vi "CompileCorrInfoNetDut.vi"(7 "Frame Direction":T1, 8 "error in (no error)":errorcluster, 10 "Frame Direction Prop":string, 11 "Device Item Ref in":T5 format="%.0x") -> (0 "error out":errorcluster, 2 "Corruption Info Network_DUT":T2 {"Frame Infos Array"."CRC Index" min=-7 max=7; "Frame Infos Array"."DLC Length  Corruption Index" min=-8 max=8}, 3 "Device Item Ref out":T5 format="%.0x")   [LabVIEW 2018, in "CAN Gateway System Explorer.lvlib"]
uses:
  CAN Gateway System Explorer.lvlib
  <vilib>/NI Veristand/Custom Device API/Custom Device Item Ref.ctl
  Shared/CTLs/Corruption Info.ctl
  Shared/CTLs/Frame.ctl
  Shared/CTLs/Signal_Data_Trigger.ctl
  Types/FrameDirection.ctl
  Types/FramesCluster.ctl
  <vilib>/NI Veristand/Custom Device API/Get Item Property (Variant).vi
  Shared/Constants.vi
  <vilib>/NI Veristand/Custom Device API/Get Item Property (String).vi
  <vilib>/NI Veristand/Custom Device API/Custom Device API.lvlib
  Shared/CAN Gateway Shared.lvlib
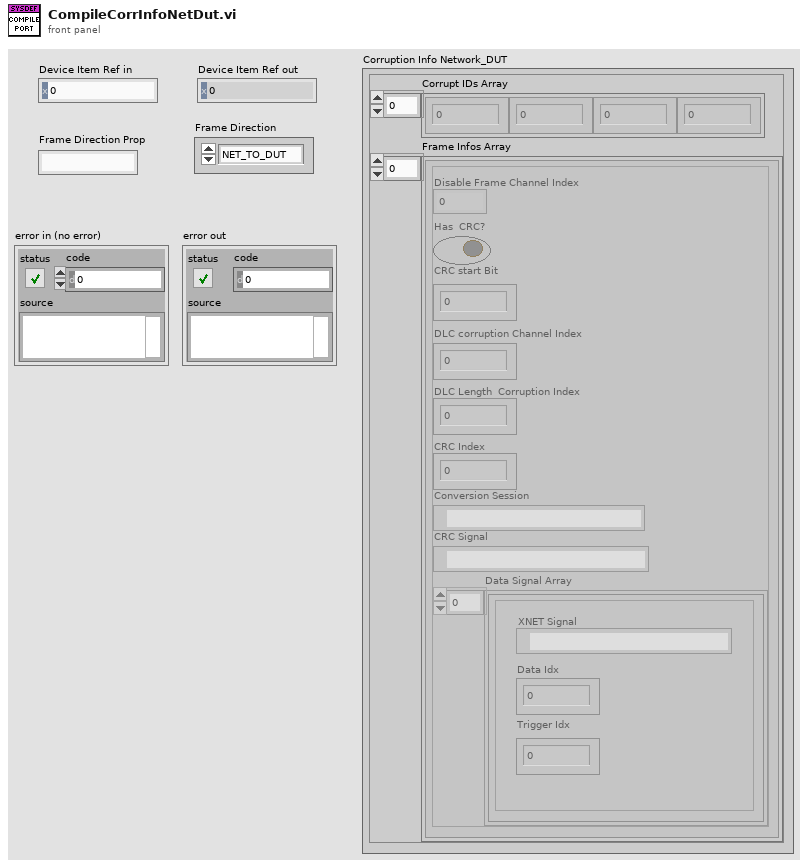
[diagram p1: front panel]
types:
  T1 = typedef "CAN Gateway System Explorer.lvlib/FrameDirection.ctl" = enum16{"NET_TO_DUT", "DUT_TO_NET"}
  T2 = typedef "CAN Gateway Shared.lvlib/Corruption Info.ctl" = cluster{"Corrupt IDs Array":u32[], "Frame Infos Array":T3[]}
  T3 = typedef "CAN Gateway Shared.lvlib/Frame.ctl" = cluster{"Disable Frame Channel Index":i32, "Has  CRC?":bool, "CRC start Bit":u32, "DLC corruption Channel Index":i32, "DLC Length  Corruption Index":i32, "CRC Index":i32, "Conversion Session":refnum<k21>, "CRC Signal":refnum<k21>, "Data Signal Array":T4[]}
  T4 = typedef "CAN Gateway Shared.lvlib/Signal_Data_Trigger.ctl" = cluster{"XNET Signal":refnum<k21>, "Data Idx":u32, "Trigger Idx":u32}
  T5 = typedef "Custom Device API.lvlib/Custom Device Item Ref.ctl" = u64
  T6 = typedef "CAN Gateway System Explorer.lvlib/FramesCluster.ctl" = cluster{"Frame":string, "Fault":bool}
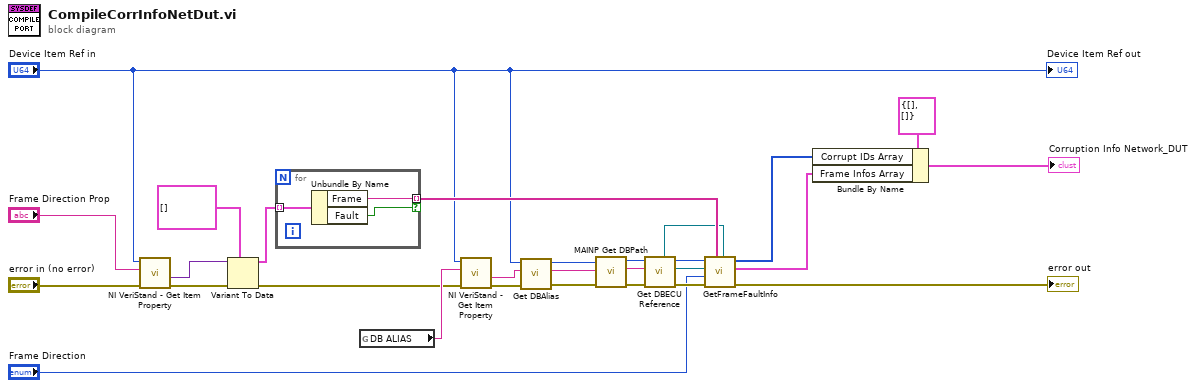
[diagram p0: block diagram]
diagram:
  n1 = call-poly <vilib>:"NI VeriStand - Get Item Property.vi"("error in (no error)"="error in (no error)", "Property Name"="Frame Direction Prop", "Item Ref in"="Device Item Ref in") -> ("error out"=w27:errorcluster, "Value"=w26:variant)  [unwired: 5 in, 2 out]
  n2 = Variant To Data(error in=w27, type=T6[] [], Variant=w26) -> (data=w24:T6[], error out=w4:errorcluster)
  n3 = for {
    tunnel: w24 -> [w31] mode=indexing
    tunnel: [w30] -> w10 mode=indexing if=w29
    n4 = Unbundle By Name(w31) -> ("Frame"=w30:string, "Fault"=w29:bool)
  }
  n5 = global read "Constants.vi" "DB ALIAS"() -> (w5:string)
  n6 = call-poly <vilib>:"NI VeriStand - Get Item Property.vi"("error in (no error)"=w4, "Property Name"=w5, "Item Ref in"="Device Item Ref in") -> ("error out"=w3:errorcluster, "Value"=w2:string)  [unwired: 5 in, 2 out]
  n7 = call "Get DBAlias.vi"("error in (no error)"=w3, "DB Alias"=w2, "Device Item Ref in"="Device Item Ref in") -> ("error out"=w22:errorcluster, "Alias"=w21:string, "Device Item Ref out"=w23:T5)  [unwired: 6 in]
  n8 = call "MAINP Get DBPath.vi"("error in (no error)"=w22, "Alias"=w21, "Device Item Ref in"=w23) -> ("error out"=w20:errorcluster, "Alias"=w18:string, "Device Item Ref out"=w19:T5)  [unwired: 5 in, 1 out]
  n9 = call "Get DBECU Reference.vi"("error in (no error)"=w20, "Alias"=w18, "Device Item Ref in"=w19) -> ("error out"=w13:errorcluster, "XNET ECU"=w12:refnum<k21>, "Device Item Ref out"=w11:T5, "XNET Cluster"=w6:refnum<k21>)  [unwired: 4 in, 1 out]
  n10 = call "GetFrameFaultInfo.vi"("XNET Cluster"=w6, "Frame Array"=w10, "error in (no error)"=w13, "Frame Direction"="Frame Direction", "ECU Reference"=w12, "Device Item Ref in"=w11) -> ("error out"=→"error out":errorcluster, "Array"=w14:T3[], "Frame ID Array"=w16:u32[])  [unwired: 3 in]
  n11 = Bundle By Name(cluster=T2 {"Corrupt IDs Array"=[], "Frame Infos Array"=[]} ("Corruption Info"), "Corrupt IDs Array"=w16, "Frame Infos Array"=w14) -> (→"Corruption Info Network_DUT":T2)
  "Device Item Ref out" <- "Device Item Ref in"
